vi "Save_AC_Data.vi"() -> (5 "Plug in titles":string[](array[string])=["AC_Data:Max:mm", "AC_Data:RMS:mm"], 7 "Plug in values":string[](array[string])=["0.000000", "NaN"])   [LabVIEW 2011]
uses:
  Globals/Meas_global.vi
  <vilib>/Analysis/5stat.llb/RMS (DBL).vi
  <vilib>/Analysis/NI_AALPro.lvlib
  <vilib>/Analysis/NI_AALBase.lvlib
panel:
  in  "Instance Name":string="RV (Vdi)"
  out "RMS":dbl[](array[numeric])=[nan, nan]
  out "Max":dbl[](array[numeric])
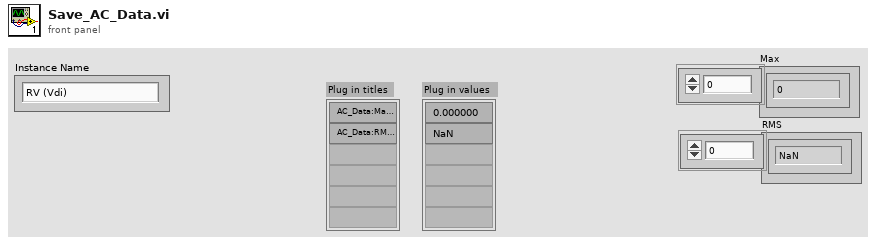
[diagram p1: front panel]
types:
  T1 = typedef "Analysis_info_cluster.ctl" = cluster{"Colour":u32, "Inst type":T2, "Inst name":string, "Symbol":string, "Code name":string, "Extra Info":string, "Inst Array":T3, "Index":i32, "Voltage Index":i32, "Extra Titles":string[], "Extra Values":string[], "Eng Values":dbl[], "Time (ms)":dbl[], "Voltage":dbl[], "U":dbl, "u^2":dbl, "u^3":dbl, "u^4":dbl, "Skew_u":dbl, "Kurt_u":dbl, "Sd Error in Mean":dbl, "% u'/U":dbl, "X":dbl, "Y":dbl, "Z":dbl, "Spectra":T4, "Autocorrelation":T4, "Timescale integral to 25%":dbl, "Sd Error in Variance":dbl, "Calib File":path, "Calib Constants":dbl[], "Histogram":T4, "Output Position":bool, "Full Stats":bool, "Weighting":dbl[]}
  T2 = typedef "Inst_type.ctl" = enum16{"Propeller anemometer", "Raw voltage", "Pressure Transducer", "Pitot-static tube", "Preston tube", "Hot wire", "Cross wire 1", "Cross wire 2", "Generic Linear", "Generic Polynomial", "Generic BackPoly", "Fast FID", "Thermocouple", "Cold wire", "Pulsed Wire", "LDA Vel", "LDA Tran time", "LDA Arr time"}
  T3 = typedef "Instrument_Array.ctl" = enum16{"PWA", "LDA", "Analogue"}
  T4 = typedef "XY_Plot_Cluster.ctl" = cluster{"First Name":string, "Second Name":string, "X axis name":string, "Y axis name":string, "X array":dbl[], "Y array":dbl[]}
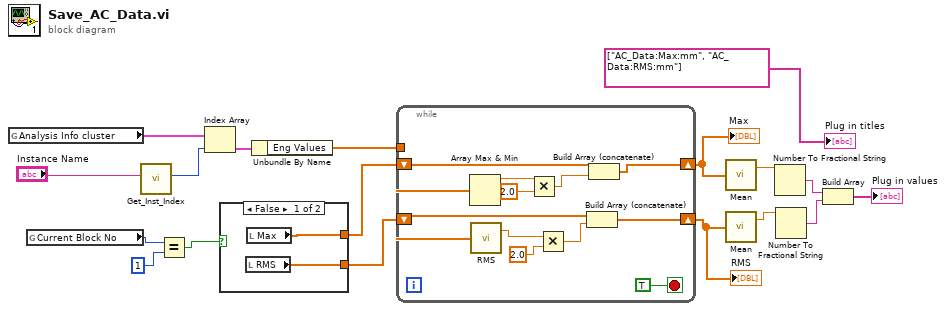
[diagram p0: block diagram]
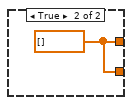
[diagram p2: hidden frame]
diagram:
  n1 = global read "Meas_global.vi" "Analysis Info cluster"() -> (w18:T1[])
  n2 = global read "Meas_global.vi" "Current Block No"() -> (w7:i32)
  n3 = call "Get_Inst_Index.vi"("Inst name search"="Instance Name") -> ("Index of Instance"=w17:i32)  [unwired: 8 in, 2 out]
  n4 = Equal?(x=w7, y=1) -> (x = y?=w5:bool)
  n5 = Index Array(array=w18, index=w17) -> (element=w16:T1)
  n6 = case shown="False" w5 {
    tunnel: [w20 w21] -> w4
    tunnel: [w19 w21] -> w2
    frame False {
      n7 = local read "RMS"() -> (w19:dbl[])
      n8 = local read "Max"() -> (w20:dbl[])
    }
    frame True {
      w21 = dbl[] []
    }
  }
  n9 = Unbundle By Name(w16) -> ("Eng Values"=w15:dbl[])
  n10 = while {
    tunnel: w15 -> [w33]
    shift-right: [w32] -> w14
    shift-left: w4 -> [w31]
    shift-right: [w30] -> w3
    shift-left: w2 -> [w29]
    stop <- TRUE stop-if-true
    n11 = Array Max & Min(array=w33) -> (max value=w27:dbl)  [unwired: 3 out]
    n12 = call-poly <vilib>:"RMS.vi"("X"=w33) -> ("rms value"=w24:dbl)  [unwired: 1 out]
    n13 = Multiply(x=w27, y=2.0) -> (x*y=w25:dbl)
    n14 = Multiply(x=w24, y=2.0) -> (x*y=w22:dbl)
    n15 = Build Array (concatenate)(w29, w22) -> (w30:dbl[])
    n16 = Build Array (concatenate)(w31, w25) -> (w32:dbl[])
  }
  "Max" <- w14
  "RMS" <- w3
  n17 = call <vilib>:"Mean.vi"("X"=w14) -> ("mean"=w12:dbl)  [unwired: 1 out]
  n18 = call <vilib>:"Mean.vi"("X"=w3) -> ("mean"=w11:dbl)  [unwired: 1 out]
  n19 = Number To Fractional String(number=w12) -> (F-format string=w10:string)  [unwired: 3 in]
  n20 = Number To Fractional String(number=w11) -> (F-format string=w9:string)  [unwired: 3 in]
  n21 = Build Array(w10, w9) -> (→"Plug in values":string[])
  "Plug in titles" <- string[] ["AC_Data:Max:mm", "AC_Data:RMS:mm"] ("Plug in titles")
